vi "Start Timer TIO.vi"(8 "error in":errorcluster) -> (0 "error out":errorcluster, 2 "Timer Cluster Out":T1, 3 "Timer task ID out":u32 format="%.0x")   [LabVIEW 2009]
uses:
  Acquisition Settings.vi
panel:
  in  "Timer Cluster":T1
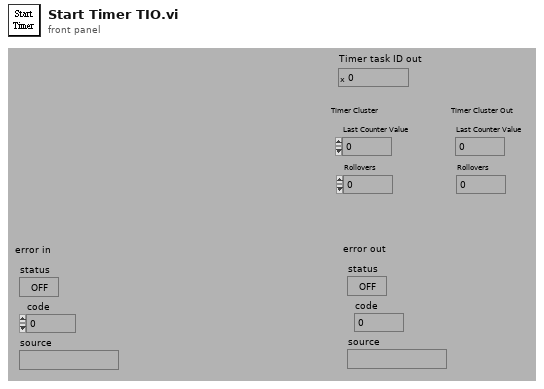
[diagram p1: front panel]
types:
  T1 = cluster{"Last Counter Value":u32, "Rollovers":i32}
  T2 = cluster{"Device Number":i16, "Counter Number":i16, "Line Type for Source":u32, "Line Number for Source":u32, "Signal Routing Configuration":i16}
  T3 = cluster{"Name":string, "Signal Routing":cluster{"signal name":u16, "signal source":u16, "signal source line number":u32, "signal name line number":u32}[]}[]
  T4 = cluster{"Name":string, "Signal Routing":cluster{"signal name":u16, "signal source":u16, "signal source line number":u32, "signal name line number":u32}[]}
  T5 = cluster{"signal name":u16, "signal source":u16, "signal source line number":u32, "signal name line number":u32}[]
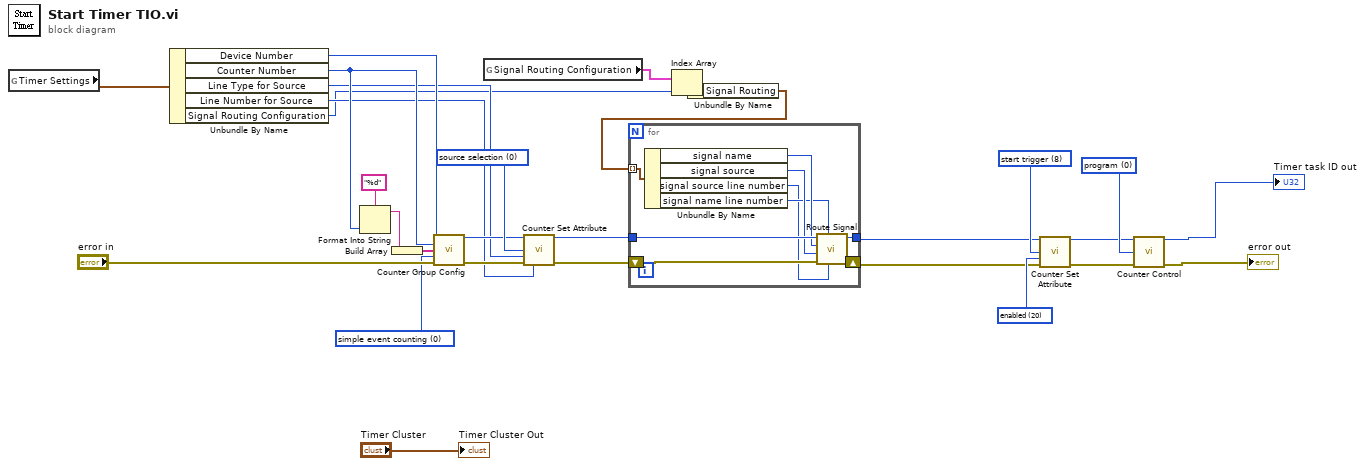
[diagram p0: block diagram]
diagram:
  w13 = u32 20 items=["yes", "no", "positive", "negative", "high", "low", "low to high", "high to low", "default", "max timebase", "other counter gate", "other counter TC", "other counter output", "other counter source", "source", "gate", "aux line", "in start trigger", "in stop trigger", "automatic", "enabled", "count up", "count down", "hardware", "single", "double", "pulse", "toggle", "quadrature encoder X1", "quadrature encoder X2", "quadrature encoder X4", "two pulse counting", "A high B high", "A high B low", "A low B high", "A low B low", "PFI n", "RTSI n", "timebase n"] ("attribute value type")
  w14 = u32 8 items=["source selection", "source polarity", "gate selection", "gate polarity", "output mode", "output polarity", "aux line selection", "aux line polarity", "start trigger", "counting synchronous", "up down", "buffer mode", "encoder type", "initial count", "pulse spec 1", "pulse spec 2", "pulse spec 3", "pulse spec 4", "auto increment", "prescale value", "Z index active", "Z index value"] ("attribute ID")
  w15 = u32 0 items=["program", "reset", "arm", "prepare", "disarm", "count up", "count down", "switch cycle", "snapshot"] ("control code")
  w18 = u32 0 items=["simple event counting", "single period measurement", "single pulse width measurement", "triggered pulse width measurement", "two signal edge separation measurement", "position measurement", "single pulse generation", "single triggered pulse generation", "retriggerable pulse generation", "pulse train generation", "frequency shift keying", "buffered event counting", "buffered period measurement", "buffered semiperiod measurement", "buffered pulse width measurement", "buffered two signal edge separation measurement", "buffered position measurement"] ("task type")
  w24 = u32 0 items=["source selection", "source polarity", "gate selection", "gate polarity", "output mode", "output polarity", "aux line selection", "aux line polarity", "start trigger", "counting synchronous", "up down", "buffer mode", "encoder type", "initial count", "pulse spec 1", "pulse spec 2", "pulse spec 3", "pulse spec 4", "auto increment", "prescale value", "Z index active", "Z index value"] ("attribute ID")
  n1 = global read "Acquisition Settings.vi" "Timer Settings"() -> (w6:T2)
  n2 = Unbundle By Name(w6) -> ("Device Number"=w25:i16, "Counter Number"=w26:i16, "Line Type for Source"=w17:u32, "Line Number for Source"=w16:u32, "Signal Routing Configuration"=w4:i16)
  n3 = Format Into String(format string="%d" ("Format String"), w26) -> (resulting string=w20:string)  [unwired: 2 in, 1 out]
  n4 = Build Array(w20) -> (w21:string[])
  n5 = call <vilib>:"Counter Group Config.vi"("device"=w25, "group"=w26, "counter list"=w21, "task type"=w18, "error in (no error)"="error in") -> ("task ID"=w23:u32, "error out"=w22:errorcluster)  [unwired: 8 in, 1 out]
  n6 = global read "Acquisition Settings.vi" "Signal Routing Configuration"() -> (w5:T3)
  n7 = call <vilib>:"Counter Set Attribute.vi"("task ID in"=w23, "attribute ID"=w24, "attribute value type"=w17, "error in (no error)"=w22, "attribute value number"=w16) -> ("task ID out"=w12:u32, "error out"=w11:errorcluster)  [unwired: 9 in]
  n8 = Index Array(array=w5, index=w4) -> (element=w3:T4)
  n9 = Unbundle By Name(w3) -> ("Signal Routing"=w2:T5)
  n10 = for {
    tunnel: w12 -> [w38]
    shift-right: [w30] -> w10
    shift-left: w11 -> [w37]
    tunnel: w2 -> [w36] mode=indexing
    tunnel: [w31] -> w9
    n11 = Unbundle By Name(w36) -> ("signal name"=w35:u16, "signal source"=w34:u16, "signal source line number"=w32:u32, "signal name line number"=w33:u32)
    n12 = call <vilib>:"Route Signal.vi"("signal source line number"=w32, "signal name line number"=w33, "error in (no error)"=w37, "signal source"=w34, "signal name"=w35, "task ID"=w38) -> ("error out"=w30:errorcluster, "task ID out"=w31:u32)  [unwired: 4 in]
  }
  n13 = call <vilib>:"Counter Set Attribute.vi"("task ID in"=w9, "attribute ID"=w14, "attribute value type"=w13, "error in (no error)"=w10) -> ("task ID out"=w8:u32, "error out"=w7:errorcluster)  [unwired: 10 in]
  n14 = call <vilib>:"Counter Control.vi"("task ID"=w8, "control code"=w15, "error in (no error)"=w7) -> ("task ID out"=→"Timer task ID out":u32, "error out"=→"error out":errorcluster)  [unwired: 11 in]
  "Timer Cluster Out" <- "Timer Cluster"
